vi "Global FieldLengthX.vi"() -> ()   [LabVIEW 2014]
panel:
  out "FieldWidthX":dbl=100.0
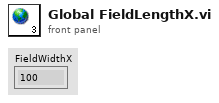
[diagram p1: front panel]
diagram:
